vi "InitSensors.vi"   [LabVIEW 2019]
doc: "This VI initializes independent sensing devices."
uses:
  <vilib>/Rock Robotics/SystemInterfaces/AI/FPGA_AIChannel.ctl
  <vilib>/Rock Robotics/WPI/ThirdParty/Phoenix-LabVIEW/Pigeon IMU/CTRE_PigeonIMU_TareType.ctl
  <vilib>/Rock Robotics/SystemInterfaces/DIO/FPGA_DIOChannel.ctl
  refnums.vi
  <vilib>/Rock Robotics/WPI/Counter/WPI_CounterDigitalInputToDigitalSource.vi
  <vilib>/Rock Robotics/WPI/Counter/WPI_CounterOpen Semi Period Mode.vi
  <vilib>/Rock Robotics/WPI/Switch/WPI_SwitchOpenLimit.vi
  <vilib>/Rock Robotics/WPI/ThirdParty/Phoenix-LabVIEW/Pigeon IMU/CTRE_PigeonIMU_Open_CAN.vi
types:
  T1 = typedef "FPGA_DIOChannel.ctl" = enum8{"DIO 0", "DIO 1", "DIO 2", "DIO 3", "DIO 4", "DIO 5", "DIO 6", "DIO 7", "DIO 8", "DIO 9", "DIO MXP 0", "DIO MXP 1", "DIO MXP 2", "DIO MXP 3", "DIO MXP 4", "DIO MXP 5", "DIO MXP 6", "DIO MXP 7", "DIO MXP 8", "DIO MXP 9", "DIO MXP 10", "DIO MXP 11", "DIO MXP 12", "DIO MXP 13", "DIO MXP 14", "DIO MXP 15", "SPI Port CS1", "SPI Port CS2", "SPI Port CS3", "SPI Port MISO", "SPI Port MOSI", "Invalid"}
  T2 = typedef "CTRE_PigeonIMU_TareType.ctl" = u8
  T3 = typedef "FPGA_AIChannel.ctl" = enum8{"AI 0", "AI 1", "AI 2", "AI 3", "AI MXP 0", "AI MXP 1", "AI MXP 2", "AI MXP 3", "Invalid"}
  T4 = typedef "WPI_SwitchDevRef.ctl" = cluster{"DevStatus":errorcluster, "DIO Channel":T1, "CntIndex":T5, "Normally Closed":bool}
  T5 = typedef "FPGA_CounterCtrSystemIndex.ctl" = enum8{"Ctr 0", "Ctr 1", "Ctr 2", "Ctr 3", "Ctr 4", "Ctr 5", "Ctr 6", "Ctr 7", "Invalid"}
  T6 = typedef "WPI_PotentiometerDevRef.ctl" = cluster{"DevStatus":errorcluster, "Analog Channel":T3, "Invert Output":bool}
  T7 = typedef "WPI_DigitalInputDevRef.ctl" = cluster{"DevStatus":errorcluster, "DIO Channel":T1}
  T8 = typedef "CTRE_PigeonIMU_DeviceRef.ctl" = cluster{"DeviceStatus":errorcluster, "Device Number":u8, "Type":T9, "Device ID":u32, "Handle":u64, "UsageFrame":u32, "Library Path":path}
  T9 = typedef "CTRE_PigeonIMU_ConnectionType.ctl" = u32
  T10 = typedef "WPI_AnalogChannelDevRef.ctl" = cluster{"DevStatus":errorcluster, "Analog Channel":T3}
  T11 = typedef "FPGA_CounterEncoderSourceConvertionLVSourceType.ctl" = cluster{"DevStatus":errorcluster, "AnalogTriggerMode?":bool, "DigitalMode":cluster{"DIO Channel":T12}, "AnalogTriggerMode":cluster{"AnalogTriggerIndex":T13, "OutputType":T14}}
  T12 = typedef "FPGA_DIODigitalSourceChannel.ctl" = enum8{"DIO 0", "DIO 1", "DIO 2", "DIO 3", "DIO 4", "DIO 5", "DIO 6", "DIO 7", "DIO 8", "DIO 9", "DIO MXP 0", "DIO MXP 1", "DIO MXP 2", "DIO MXP 3", "DIO MXP 4", "DIO MXP 5", "DIO MXP 6", "DIO MXP 7", "DIO MXP 8", "DIO MXP 9", "DIO MXP 10", "DIO MXP 11", "DIO MXP 12", "DIO MXP 13", "DIO MXP 14", "DIO MXP 15", "SPI Port CS1", "SPI Port CS2", "SPI Port CS3", "SPI Port MISO", "SPI Port MOSI", "Disabled"}
  T13 = typedef "FPGA_AnalogTriggerIndex.ctl" = enum8{"Trig 0", "Trig 1", "Trig 2", "Trig 3", "Trig 4", "Trig 5", "Trig 6", "Trig 7", "Invalid"}
  T14 = typedef "FPGA_AnalogTriggerOutType.ctl" = enum16{"InWindow", "TriggerState", "Rising", "Falling"}
  T15 = typedef "WPI_CounterDevRef.ctl" = cluster{"DevStatus":errorcluster, "CntIndex":T5}
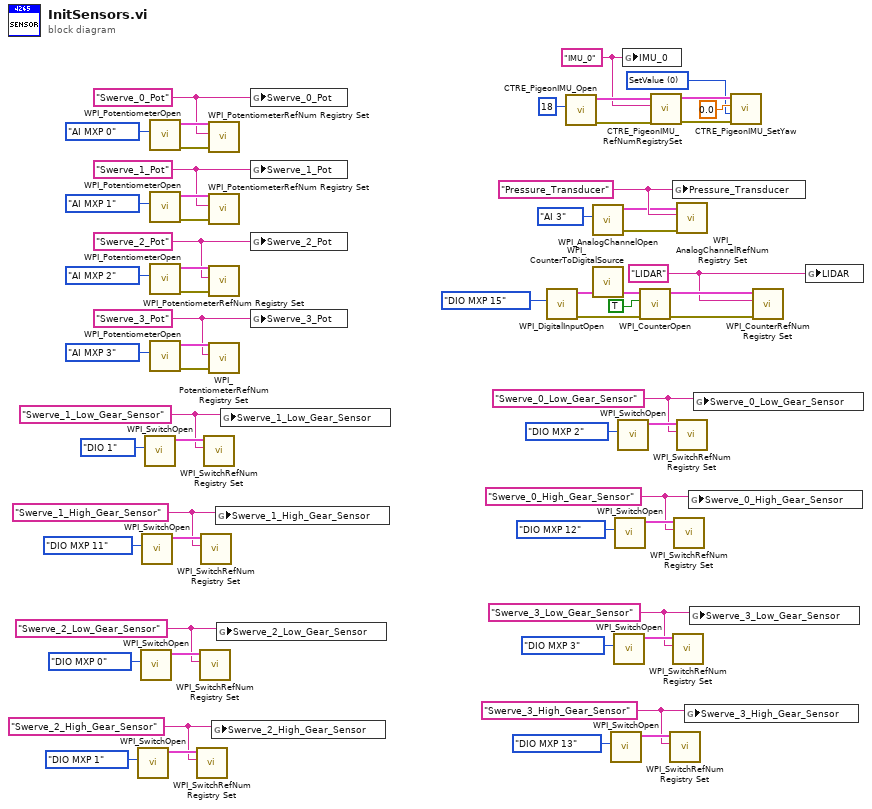
[diagram p0: block diagram]
diagram:
  w2 = "Swerve_2_High_Gear_Sensor" ("refnum name")
  w5 = "Swerve_2_Low_Gear_Sensor" ("refnum name")
  w8 = "Swerve_3_High_Gear_Sensor" ("refnum name")
  w11 = "Swerve_3_Low_Gear_Sensor" ("refnum name")
  w14 = "Swerve_1_High_Gear_Sensor" ("refnum name")
  w17 = "Swerve_1_Low_Gear_Sensor" ("refnum name")
  w20 = "Swerve_0_High_Gear_Sensor" ("refnum name")
  w23 = "Swerve_0_Low_Gear_Sensor" ("refnum name")
  w26 = "LIDAR" ("refnum name")
  w34 = T2 0 items=["SetValue"=0, "AddOffset"=1, "MatchCompass"=2, "SetOffset"=255] ("TareType (SetValue)")
  w38 = "IMU_0" ("refnum name")
  w43 = "Pressure_Transducer" ("Pressure_Transducer")
  w49 = "Swerve_3_Pot"
  w52 = "Swerve_2_Pot"
  w55 = "Swerve_1_Pot"
  w58 = "Swerve_0_Pot"
  n1 = call-poly <vilib>:"WPI_SwitchOpen.vi"("DIO Channel"=FPGA_DIOChannel."DIO MXP 1") -> ("SwitchDevRef"=w3:T4)  [unwired: 9 in, 1 out]
  n2 = call-poly <vilib>:"WPI_SwitchOpen.vi"("DIO Channel"=FPGA_DIOChannel."DIO MXP 0") -> ("SwitchDevRef"=w6:T4)  [unwired: 9 in, 1 out]
  n3 = call-poly <vilib>:"WPI_SwitchOpen.vi"("DIO Channel"=FPGA_DIOChannel."DIO MXP 11") -> ("SwitchDevRef"=w15:T4)  [unwired: 9 in, 1 out]
  n4 = call-poly <vilib>:"WPI_SwitchOpen.vi"("DIO Channel"=FPGA_DIOChannel."DIO 1") -> ("SwitchDevRef"=w18:T4)  [unwired: 9 in, 1 out]
  n5 = call <vilib>:"WPI_PotentiometerOpen.vi"("Analog Channel"=FPGA_AIChannel."AI MXP 0") -> ("error out"=w48:errorcluster, "PotDevRef"=w60:T6)  [unwired: 9 in]
  n6 = call <vilib>:"WPI_PotentiometerOpen.vi"("Analog Channel"=FPGA_AIChannel."AI MXP 1") -> ("error out"=w47:errorcluster, "PotDevRef"=w57:T6)  [unwired: 9 in]
  n7 = call <vilib>:"WPI_PotentiometerOpen.vi"("Analog Channel"=FPGA_AIChannel."AI MXP 2") -> ("error out"=w46:errorcluster, "PotDevRef"=w54:T6)  [unwired: 9 in]
  n8 = call <vilib>:"WPI_PotentiometerOpen.vi"("Analog Channel"=FPGA_AIChannel."AI MXP 3") -> ("error out"=w45:errorcluster, "PotDevRef"=w51:T6)  [unwired: 9 in]
  n9 = call <vilib>:"WPI_SwitchRefNum Registry Set.vi"("refnum name"=w2, "SwitchDevRef"=w3) -> ()  [unwired: 8 in, 2 out]
  n10 = call <vilib>:"WPI_SwitchRefNum Registry Set.vi"("refnum name"=w5, "SwitchDevRef"=w6) -> ()  [unwired: 8 in, 2 out]
  n11 = call <vilib>:"WPI_SwitchRefNum Registry Set.vi"("refnum name"=w14, "SwitchDevRef"=w15) -> ()  [unwired: 8 in, 2 out]
  n12 = call <vilib>:"WPI_SwitchRefNum Registry Set.vi"("refnum name"=w17, "SwitchDevRef"=w18) -> ()  [unwired: 8 in, 2 out]
  n13 = call <vilib>:"WPI_PotentiometerRefNum Registry Set.vi"("error in (no error)"=w48, "refnum name"=w58, "PotDevRef"=w60) -> ()  [unwired: 7 in, 2 out]
  n14 = call <vilib>:"WPI_PotentiometerRefNum Registry Set.vi"("error in (no error)"=w47, "refnum name"=w55, "PotDevRef"=w57) -> ()  [unwired: 7 in, 2 out]
  n15 = call <vilib>:"WPI_PotentiometerRefNum Registry Set.vi"("error in (no error)"=w46, "refnum name"=w52, "PotDevRef"=w54) -> ()  [unwired: 7 in, 2 out]
  n16 = call <vilib>:"WPI_PotentiometerRefNum Registry Set.vi"("error in (no error)"=w45, "refnum name"=w49, "PotDevRef"=w51) -> ()  [unwired: 7 in, 2 out]
  n17 = global write "refnums.vi" "Swerve_2_High_Gear_Sensor"(w2) -> ()
  n18 = global write "refnums.vi" "Swerve_1_High_Gear_Sensor"(w14) -> ()
  n19 = global write "refnums.vi" "Swerve_2_Low_Gear_Sensor"(w5) -> ()
  n20 = global write "refnums.vi" "Swerve_1_Low_Gear_Sensor"(w17) -> ()
  n21 = global write "refnums.vi" "Swerve_0_Pot"(w58) -> ()
  n22 = global write "refnums.vi" "Swerve_1_Pot"(w55) -> ()
  n23 = global write "refnums.vi" "Swerve_2_Pot"(w52) -> ()
  n24 = global write "refnums.vi" "Swerve_3_Pot"(w49) -> ()
  n25 = call <vilib>:"WPI_DigitalInputOpen.vi"("DIO Channel"=FPGA_DIOChannel."DIO MXP 15" ("Source")) -> ("error out"=w29:errorcluster, "DigitalInputDevRef"=w31:T7)  [unwired: 1 in, 8 out]
  n26 = call-poly <vilib>:"CTRE_PigeonIMU_Open.vi"("Device Number"=u8 18) -> ("error out"=w39:errorcluster, "PigeonIMUDevRef"=w40:T8)  [unwired: 9 in]
  n27 = call <vilib>:"WPI_AnalogChannelOpen.vi"("Analog Channel"=FPGA_AIChannel."AI 3") -> ("error out"=w41:errorcluster, "AIDeviceRef"=w42:T10)  [unwired: 9 in]
  n28 = call-poly <vilib>:"WPI_CounterToDigitalSource.vi"("DigitalInputDevRef"=w31) -> ("Digital Source"=w33:T11)  [unwired: 6 out]
  n29 = call-poly <vilib>:"WPI_SwitchOpen.vi"("DIO Channel"=FPGA_DIOChannel."DIO MXP 13") -> ("SwitchDevRef"=w9:T4)  [unwired: 9 in, 1 out]
  n30 = call-poly <vilib>:"WPI_SwitchOpen.vi"("DIO Channel"=FPGA_DIOChannel."DIO MXP 3") -> ("SwitchDevRef"=w12:T4)  [unwired: 9 in, 1 out]
  n31 = call-poly <vilib>:"WPI_SwitchOpen.vi"("DIO Channel"=FPGA_DIOChannel."DIO MXP 12") -> ("SwitchDevRef"=w21:T4)  [unwired: 9 in, 1 out]
  n32 = call-poly <vilib>:"WPI_SwitchOpen.vi"("DIO Channel"=FPGA_DIOChannel."DIO MXP 2") -> ("SwitchDevRef"=w24:T4)  [unwired: 9 in, 1 out]
  n33 = global write "refnums.vi" "IMU_0"(w38) -> ()
  n34 = call-poly <vilib>:"WPI_CounterOpen.vi"("error in (no error)"=w29, "High Pulse (T)"=TRUE, "Source"=w33) -> ("error out"=w28:errorcluster, "CounterDevRef"=w30:T15)  [unwired: 2 in, 5 out]
  n35 = call <vilib>:"CTRE_PigeonIMU_RefNumRegistrySet.vi"("error in (no error)"=w39, "refnum name"=w38, "PigeonIMUDevRef"=w40) -> ("error out"=w36:errorcluster, "PigeonIMUDevRef"=w37:T8)  [unwired: 7 in]
  n36 = call <vilib>:"WPI_SwitchRefNum Registry Set.vi"("refnum name"=w8, "SwitchDevRef"=w9) -> ()  [unwired: 8 in, 2 out]
  n37 = global write "refnums.vi" "Pressure_Transducer"(w43) -> ()
  n38 = call <vilib>:"WPI_SwitchRefNum Registry Set.vi"("refnum name"=w11, "SwitchDevRef"=w12) -> ()  [unwired: 8 in, 2 out]
  n39 = call <vilib>:"WPI_SwitchRefNum Registry Set.vi"("refnum name"=w20, "SwitchDevRef"=w21) -> ()  [unwired: 8 in, 2 out]
  n40 = call <vilib>:"WPI_AnalogChannelRefNum Registry Set.vi"("error in (no error)"=w41, "refnum name"=w43, "AIDeviceRef"=w42) -> ()  [unwired: 7 in, 2 out]
  n41 = call <vilib>:"WPI_SwitchRefNum Registry Set.vi"("refnum name"=w23, "SwitchDevRef"=w24) -> ()  [unwired: 8 in, 2 out]
  n42 = global write "refnums.vi" "Swerve_3_High_Gear_Sensor"(w8) -> ()
  n43 = global write "refnums.vi" "Swerve_0_High_Gear_Sensor"(w20) -> ()
  n44 = global write "refnums.vi" "Swerve_3_Low_Gear_Sensor"(w11) -> ()
  n45 = global write "refnums.vi" "Swerve_0_Low_Gear_Sensor"(w23) -> ()
  n46 = call <vilib>:"CTRE_PigeonIMU_SetYaw.vi"("error in (no error)"=w36, "TareType (SetValue)"=w34, "Value"=0.0, "PigeonIMUDevRef"=w37) -> ()  [unwired: 6 in, 2 out]
  n47 = call <vilib>:"WPI_CounterRefNum Registry Set.vi"("error in (no error)"=w28, "refnum name"=w26, "CounterDevRef"=w30) -> ()  [unwired: 7 in, 2 out]
  n48 = global write "refnums.vi" "LIDAR"(w26) -> ()
